vi "Test Process Helper Loop Stopped when Process Stopped.vi"(8 "error in (no error)":errorcluster, 11 "Helper Loop Test In":refnum<class "Process Dev Test.lvclass">) -> (0 "error out":errorcluster, 3 "Helper Loop Test Out":refnum<class "Process Dev Test.lvclass">)   [LabVIEW 2020, in "Process Dev Test.lvclass"]
uses:
  Process Dev Test.lvclass
  C:/Program Files (x86)/National Instruments/LabVIEW 2020/vi.lib/Astemes/LUnit/Test Case.lvclass
  source/Framework Test Suite/Mock Process/Mock Process.lvclass
  C:/Git/triarc-framework/source/Framework/Process/Process.lvclass
  source/Framework/Process/Process.lvclass/Process.ctl
  <vilib>/Astemes/LUnit/Test Case.lvclass/Test Case.ctl
  <vilib>/Astemes/LUnit/LUnit Assertion Result.lvclass/LUnit Assertion Result.ctl
  <vilib>/Astemes/LUnit/LUnit Test Case Result.lvclass/LUnit Test Case Result.ctl
  <vilib>/Astemes/LUnit/LUnit Method Result.lvclass/LUnit Method Result.ctl
  4331ba45-8b7f-4b93-ba6e-ee1d1159701a.vi
  0f3fef22-4207-48e1-9b8b-17390fd24f63.vi
  e1ea3113-d8f4-4be9-9a25-bccd302f8800.vi
  source/Framework/Process/Public/Lifecycle/Get Lifecycle State.vi
  source/Framework/Broadcast Event Helpers/Dequeue Broadcast Message by Message Cluster.vi
  <vilib>/Astemes/LUnit/Palette/Pass.vi
  <vilib>/Astemes/LUnit/Palette/Fail.vi
  <vilib>/Astemes/LUnit/Compare Variants.vi
  <vilib>/Astemes/LUnit/Describe Comparison.vi
  <vilib>/Astemes/LUnit/Set Assertion Type.vi
  source/Framework/Process/Private/SubVIs/Wait for finish.vi
  source/Framework/Process/Protected/Messaging/Enqueue Message.vi
  source/Framework/Process/Private/SubVIs/Set Lifecycle State.vi
  <vilib>/Utility/error.llb/Clear Errors.vi
  source/Framework/Broadcast Event Helpers/Execution timer.vi
  <vilib>/Astemes/LUnit/Add test result.vi
  <vilib>/Astemes/LUnit/LUnit Write Passed.vi
  <vilib>/Astemes/LUnit/LUnit Write Message.vi
  <vilib>/Astemes/LUnit/LUnit Write Description.vi
  <vilib>/Astemes/LUnit/Variant to string.vi
  <vilib>/Astemes/LUnit/LUnit Write Assertion Type.vi
  source/Framework/Process/Private/SubVIs/Handle Debug Data.vi
  <vilib>/Astemes/LUnit/LUnit Record Assertion Result.vi
  source/Framework/Logging/Log Debug.vi
  <vilib>/AdvancedString/1D String Array to Delimited String.vi
  <vilib>/Utility/High Resolution Relative Seconds.vi
  <vilib>/Astemes/LUnit/LUnit Aggregate Assertion Results.vi
  <vilib>/Astemes/LUnit/Assertion Result/LUnit Read Status.vi
  <vilib>/Astemes/LUnit/LUnit Read Message.vi
  <vilib>/Astemes/LUnit/LUnit Read Description.vi
  <vilib>/Astemes/LUnit/Method Result/LUnit Merge Status.vi
  <vilib>/Astemes/LUnit/LUnit Concatenate result strings.vi
  <vilib>/Utility/error.llb/Error Cluster From Error Code.vi
  source/Framework/Broadcast Event Helpers/Dequeue Broadcast Message.vi
  <vilib>/Utility/Data Type/Get Type Information.vi
  <vilib>/Utility/LVClass/Get LV Class Name.vi
  source/Framework/Process/Public/Read Name.vi
  <vilib>/Astemes/LUnit/LUnit Assertion Result.lvclass
  source/Framework/Process/Process.lvclass
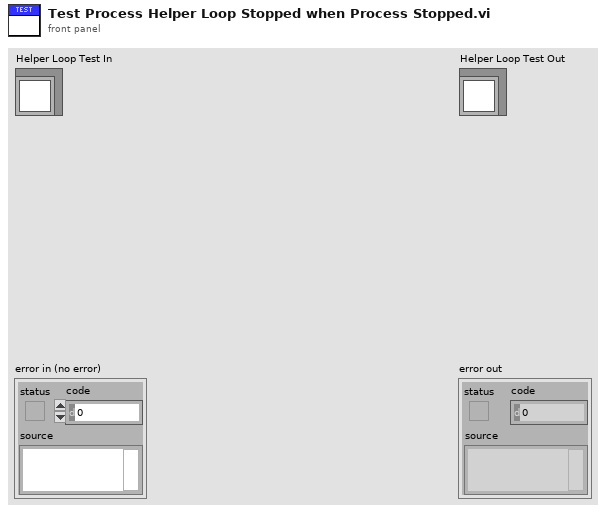
[diagram p1: front panel]
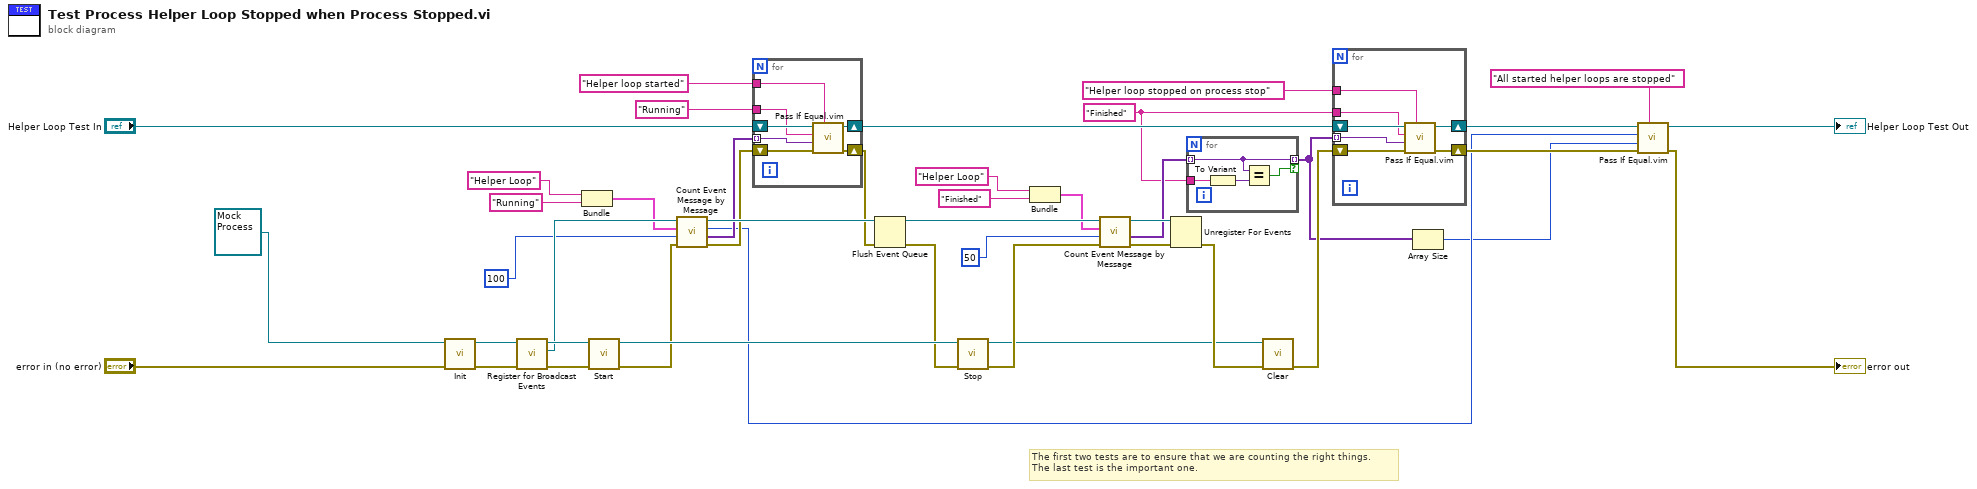
[diagram p0: block diagram]
diagram:
  w9 = "Finished" ("Description")
  # "The first two tests are to ensure that we are counting the right things. \nThe last test is the important one."
  n1 = call-dynamic "Init.vi"("error in (no error)"="error in (no error)", "Mock Process In"=refnum<class "Mock Process.lvclass"> refnum ("Mock Process.lvclass")) -> ("error out"=w38:errorcluster, "Mock Process Out"=w39:refnum<class "Mock Process.lvclass">)  [unwired: 8 in]
  n2 = call "Register for Broadcast Events.vi"("error in (no error)"=w38, "Process In"=w39) -> ("error out"=w36:errorcluster, "Event Registration Refnum Out"=w26:refnum<event-registration>, "Process Out"=w37:refnum<class "Mock Process.lvclass">)  [unwired: 7 in]
  n3 = Bundle("y"="Helper Loop", "Description"="Running") -> (w6:cluster{"y":string, "Description":string})  [unwired: 1 in]
  n4 = call "Start.vi"("error in (no error)"=w36, "Process In"=w37) -> ("error out"=w24:errorcluster, "Process Out"=w35:refnum<class "Mock Process.lvclass">)  [unwired: 7 in, 1 out]
  n5 = call "Count Event Message by Message.vi"("error in (no error)"=w24, "Timeout"=100 ("Timeout (-1)"), "Message"=w6, "Event Registration Refnum in"=w26) -> ("error out"=w20:errorcluster, "Message Data"=w16:variant[], "Count"=w12:i32, "Event Registration Refnum out"=w25:refnum<event-registration>)  [unwired: 4 in]
  n6 = for {
    tunnel: "Helper loop started" ("Description") -> [w47]
    tunnel: "Running" ("Description") -> [w46]
    shift-right: [w51] -> w22
    shift-left: "Helper Loop Test In" -> [w50]
    shift-right: [w48] -> w19
    shift-left: w20 -> [w49]
    tunnel: w16 -> [w45] mode=indexing
    n7 = call "Pass If Equal.vim"("Description"=w47, "error in (no error)"=w49, "Actual"=w45, "Expected"=w46, "LUnit Test Case In"=w50) -> ("error out"=w48:errorcluster, "LUnit Test Case Out"=w51:refnum<class "Process Dev Test.lvclass">)  [unwired: 5 in]
  }
  n8 = Flush Event Queue(0:w25, 3:w19) -> (8:w31:refnum<event-registration>, 11:w30:errorcluster)  [unwired: 4 in, 1 out]
  n9 = call "Stop.vi"("error in (no error)"=w30, "Process In"=w35) -> ("error out"=w29:errorcluster, "Process Out"=w28:refnum<class "Mock Process.lvclass">)  [unwired: 7 in, 1 out]
  n10 = Bundle("y"="Helper Loop", "Description"="Finished") -> (w2:cluster{"y":string, "Description":string})  [unwired: 1 in]
  n11 = call "Count Event Message by Message.vi"("error in (no error)"=w29, "Timeout"=50 ("Timeout (-1)"), "Message"=w2, "Event Registration Refnum in"=w31) -> ("error out"=w27:errorcluster, "Message Data"=w10:variant[], "Event Registration Refnum out"=w33:refnum<event-registration>)  [unwired: 4 in, 1 out]
  n12 = Unregister For Events(event registration refnum=w33, error in=w27) -> (error out=w32:errorcluster)
  n13 = for {
    tunnel: [w52] -> w8 mode=indexing if=w54
    tunnel: w9 -> [w53]
    tunnel: w10 -> [w52] mode=indexing
    n14 = To Variant(anything=w53) -> (Variant=w55:variant)
    n15 = Equal?(x=w52, y=w55) -> (x = y?=w54:bool)
  }
  n16 = call-dynamic "Clear.vi"("error in (no error)"=w32, "Mock Process In"=w28) -> ("error out"=w34:errorcluster)  [unwired: 9 in]
  n17 = for {
    tunnel: w8 -> [w59] mode=indexing
    shift-right: [w60] -> w13
    shift-left: w34 -> [w62]
    shift-right: [w61] -> w14
    shift-left: w22 -> [w58]
    tunnel: "Helper loop stopped on process stop" ("Description") -> [w57]
    tunnel: w9 -> [w56]
    n18 = call "Pass If Equal.vim"("Description"=w57, "error in (no error)"=w62, "Actual"=w59, "Expected"=w56, "LUnit Test Case In"=w58) -> ("error out"=w60:errorcluster, "LUnit Test Case Out"=w61:refnum<class "Process Dev Test.lvclass">)  [unwired: 5 in]
  }
  n19 = Array Size(array=w8) -> (size(s)=w7:i32)
  n20 = call "Pass If Equal.vim"("Description"="All started helper loops are stopped", "error in (no error)"=w13, "Actual"=w7, "Expected"=w12, "LUnit Test Case In"=w14) -> ("error out"=→"error out":errorcluster, "LUnit Test Case Out"=→"Helper Loop Test Out":refnum<class "Process Dev Test.lvclass">)  [unwired: 5 in]
